vi "DIHB DAQmx Task Name - Constant.vi"() -> (3 "DIHB DAQmx Task Name":string)   [LabVIEW 2020]
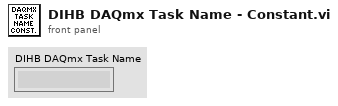
[diagram p1: front panel]
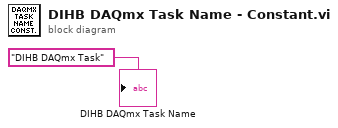
[diagram p0: block diagram]
diagram:
  "DIHB DAQmx Task Name" <- "DIHB DAQmx Task" ("new task name")
